vi "set up complex region.vi"(7 "scale factor":dbl=1.0, 11 "z in window":cdb[](array[numeric])) -> (0 "z  normalized":cdb[](array[numeric]), 1 "normalization factor":dbl=1.0, 2 "data center":cdb, 3 "complex region":T1)   [LabVIEW 2015]
uses:
  complex region.ctl
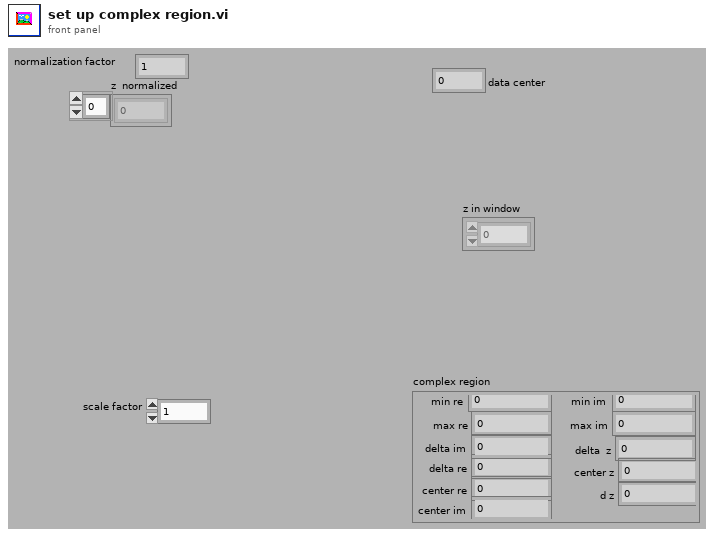
[diagram p1: front panel]
types:
  T1 = typedef "complex region.ctl" = cluster{"max re":dbl, "min re":dbl, "max im":dbl, "min im":dbl, "delta re":dbl, "delta im":dbl, "center re":dbl, "delta  z":cdb, "center im":dbl, "center z":cdb, "d im":dbl, "d re":dbl, "d z":cdb}
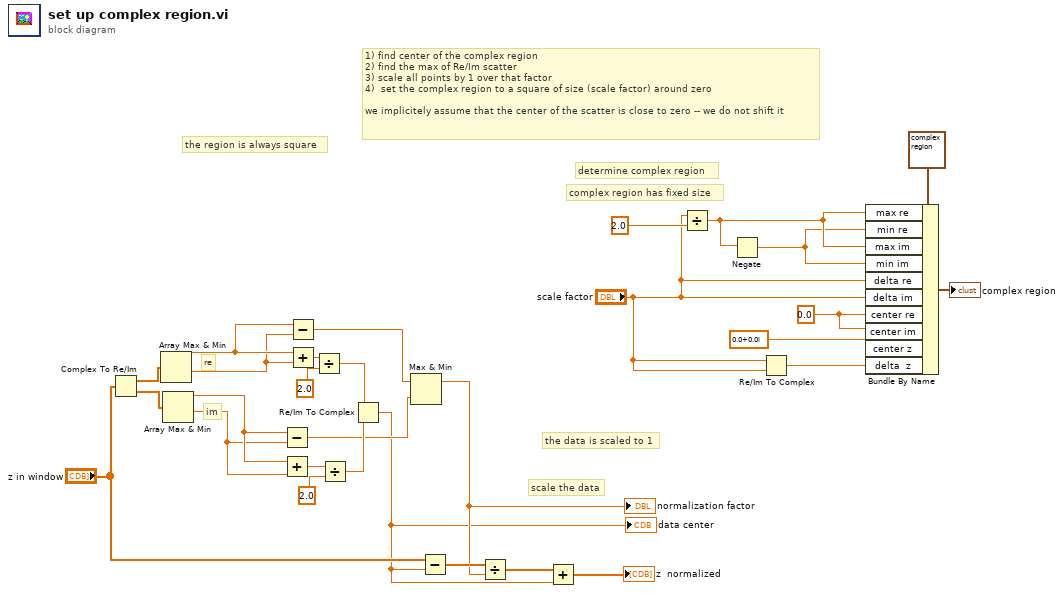
[diagram p0: block diagram]
diagram:
  w8 = 0.0
  # "the data is scaled to 1"
  # "complex region has fixed size"
  # "scale the data"
  # "1) find center of the complex region\n2) find the max of Re/Im scatter \n3) scale all points by 1 over that factor\n4)  set the complex region to a square of size (scale factor) around zero\n\nwe implicitely assume that the center of the scatter is close to zero -- we do not shift it"
  # "the region is always square"
  # "determine complex region"
  # "im"
  # "re"
  n1 = Complex To Re/Im(x + iy="z in window") -> (x=w25:dbl[], y=w24:dbl[])
  n2 = Array Max & Min(array=w25) -> (max value=w20:dbl, min value=w19:dbl)  [unwired: 2 out]
  n3 = Array Max & Min(array=w24) -> (max value=w23:dbl, min value=w22:dbl)  [unwired: 2 out]
  n4 = Subtract(x=w23, y=w22) -> (x-y=w13:dbl)
  n5 = Add(x=w23, y=w22) -> (x+y=w21:dbl)
  n6 = Subtract(x=w20, y=w19) -> (x-y=w14:dbl)
  n7 = Add(x=w20, y=w19) -> (x+y=w18:dbl)
  n8 = Divide(x=w18, y=2.0) -> (x/y=w16:dbl)
  n9 = Divide(x=w21, y=2.0) -> (x/y=w15:dbl)
  n10 = Re/Im To Complex(1:w15, 2:w16) -> (0:w2:cdb)
  "data center" <- w2
  n11 = Max & Min(x=w14, y=w13) -> (max(x,y)=w4:dbl)  [unwired: 1 out]
  "normalization factor" <- w4
  n12 = Subtract(x="z in window", y=w2) -> (x-y=w5:cdb[])
  n13 = Divide(x=w5, y=w4) -> (x/y=w3:cdb[])
  n14 = Add(x=w3, y=w2) -> (x+y=→"z  normalized":cdb[])
  n15 = Divide(x="scale factor", y=2.0) -> (x/y=w11:dbl)
  n16 = Negate(x=w11) -> (-x=w10:dbl)
  n17 = Re/Im To Complex(1:"scale factor", 2:"scale factor") -> (0:w17:cdb)
  n18 = Bundle By Name(cluster=T1 {"max re"=0.0, "min re"=0.0, "max im"=0.0, "min im"=0.0, "delta re"=0.0, "delta im"=0.0, "center re"=0.0, "delta  z"=0.0+0.0i, "center im"=0.0, "center z"=0.0+0.0i, "d im"=0.0, "d re"=0.0, "d z"=0.0+0.0i} ("complex region"), "max re"=w11, "min re"=w10, "max im"=w11, "min im"=w10, "delta re"="scale factor", "delta im"="scale factor", "center re"=w8, "center im"=w8, "center z"=cdb 0.0+0.0i ("x + iy"), "delta  z"=w17) -> (→"complex region":T1)
